vi "CalculateBounds.vi"(7 "menu in":refnum<class "menu.lvclass">, 8 "error in (no error)":errorcluster, 11 "separator item in":refnum<class "separator item.lvclass">) -> (0 "error out":errorcluster, 2 "bounds":cluster{"width":u32, "height":u32}, 3 "separator item out":refnum<class "separator item.lvclass">)   [LabVIEW 2009, in "separator item.lvclass"]
uses:
  separator item.lvclass
  Menu/menu.lvclass
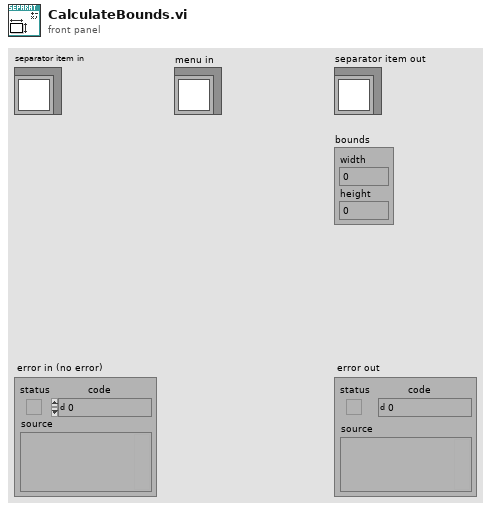
[diagram p1: front panel]
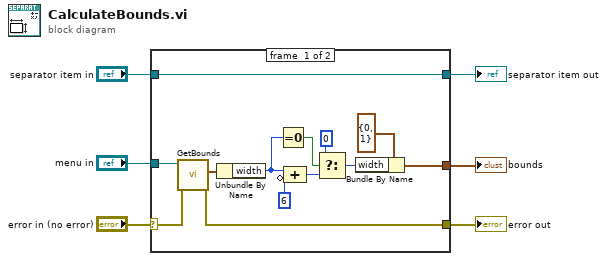
[diagram p0: block diagram]
diagram:
  n1 = case shown="No Error" "error in (no error)" {
    selector: "error in (no error)" -> [w17 w21]
    tunnel: [w16 w21] -> w3
    tunnel: [w19 w20] -> w5
    tunnel: "separator item in" -> [w19 w20]
    tunnel: "menu in" -> [w18 _]
    tunnel: [w12 _] -> w1
    frame #0 {
      n2 = call "GetBounds.vi"("error in (no error)"=w17, "menu in"=w18) -> ("error out"=w16:errorcluster, "bounds"=w14:cluster{"width":u32, "height":u32})  [unwired: 7 in, 1 out]
      n3 = Unbundle By Name(w14) -> ("width"=w11:u32)
      n4 = Equal To 0?(x=w11) -> (x = 0?=w8:bool)
      n5 = Compound Arithmetic op=ADD(w11, invert u32 6 ("height")) -> (w10:u32)
      n6 = Select(t=u32 0 ("width"), s=w8, f=w10) -> (s? t:f=w9:u32)
      n7 = Bundle By Name(cluster=cluster{"width":u32, "height":u32} {"width"=0, "height"=1} ("bounds"), "width"=w9) -> (w12:cluster{"width":u32, "height":u32})
    }
    frame #1 {
    }
  }
  "separator item out" <- w5
  "error out" <- w3
  "bounds" <- w1
